vi "质控启动器.vi"(8 "error in (no error)":errorcluster, 9 "加标体积":sgl, 10 "流程控制":T1, 11 "Slave ID":T2) -> (0 "error out":errorcluster)   [LabVIEW 2016, in "质控单元V1.lvlib"]
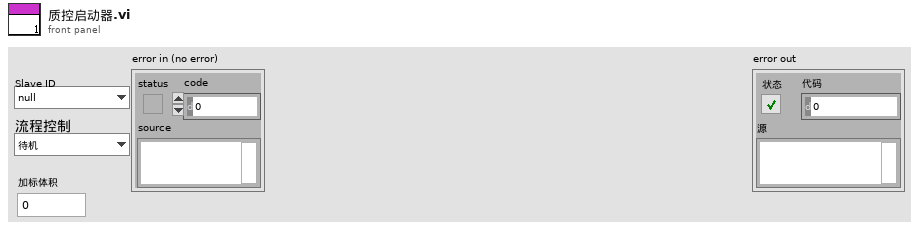
[diagram p1: front panel]
types:
  T1 = typedef "质控单元V1.lvlib/质控标准流程.ctl" = enum16{"待机", "启动进样流程", "启动加标流程", "启动排液流程", "启动水样润洗流程", "启动加标润洗流程", "停止流程", "启动搅拌流程", "停止搅拌流程"}
  T2 = typedef "质控单元V1.lvlib/质控slave id.ctl" = enum16{"null", "氨氮", "总磷", "CODMn", "CODCr", "总氮"}
  T3 = typedef "质控单元V1.lvlib/质控流程控制.ctl" = enum16{"待机", "润洗", "进样", "加标", "排液", "搅拌"}
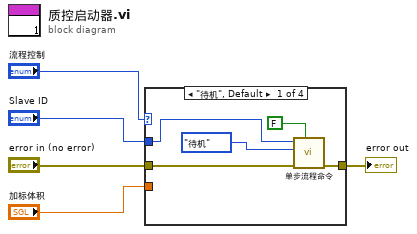
[diagram p0: block diagram]
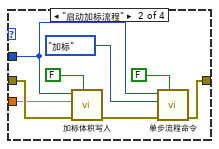
[diagram p2: hidden frame]
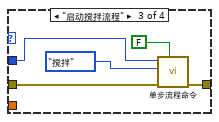
[diagram p3: hidden frame]
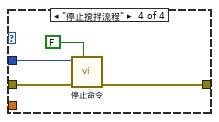
[diagram p4: hidden frame]
diagram:
  n1 = case shown="\"待机\", Default" "流程控制" {
    tunnel: "Slave ID" -> [w10 w13 w23 w27]
    tunnel: [w8 w14 w21 w25] -> w1
    tunnel: "error in (no error)" -> [w7 w17 w22 w26]
    tunnel: "加标体积" -> [_ w16 _ _]
    frame "待机", Default {
      n2 = call "单步流程命令.vi"("是否启用通讯通知"=FALSE, "error in (no error)"=w7, "流程控制"=质控流程控制."待机", "Slave ID"=w10) -> ("error out"=w8:errorcluster)  [unwired: 7 in]
    }
    frame "启动加标流程" {
      n3 = call "加标体积写入.vi"("是否启用通讯通知"=FALSE, "error in (no error)"=w17, "加标体积"=w16, "Slave ID"=w13) -> ("error out"=w15:errorcluster)  [unwired: 7 in]
      n4 = call "单步流程命令.vi"("是否启用通讯通知"=FALSE, "error in (no error)"=w15, "流程控制"=质控流程控制."加标", "Slave ID"=w13) -> ("error out"=w14:errorcluster)  [unwired: 7 in]
    }
    frame "启动搅拌流程" {
      n5 = call "单步流程命令.vi"("是否启用通讯通知"=FALSE, "error in (no error)"=w22, "流程控制"=质控流程控制."搅拌", "Slave ID"=w23) -> ("error out"=w21:errorcluster)  [unwired: 7 in]
    }
    frame "停止搅拌流程" {
      n6 = call "停止命令.vi"("是否启用通讯通知"=FALSE, "error in (no error)"=w26, "Slave ID"=w27) -> ("error out"=w25:errorcluster)  [unwired: 8 in]
    }
  }
  "error out" <- w1
